vi "Change Current.vi"() -> ()   [LabVIEW 2011]
uses:
  <instrlib>/BK Precision 85XX Series/BK Precision 85XX Series.lvlib
panel:
  in  "CC Current (0)":dbl
  in  "VISA resource name":refnum<visa-resource-name>
  # "A"
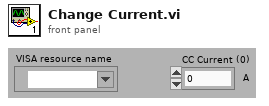
[diagram p1: front panel]
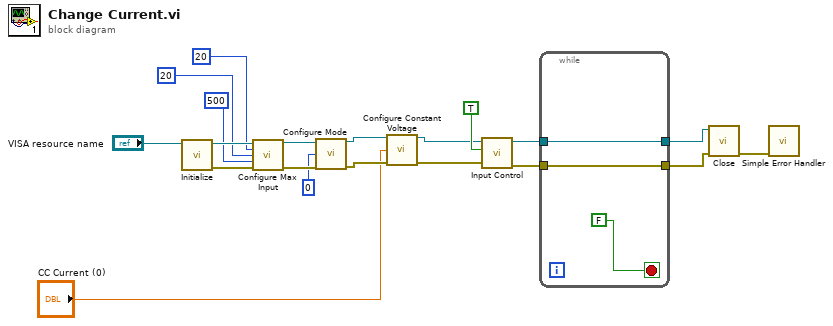
[diagram p0: block diagram]
diagram:
  n1 = call <instrlib>:"Initialize.vi"("VISA resource name"="VISA resource name") -> ("error out"=w20:errorcluster, "VISA resource name out"=w16:refnum<visa-resource-name>)  [unwired: 9 in]
  n2 = call <instrlib>:"Configure Max Input.vi"("VISA resource name"=w16, "Maximum Input Voltage (0)"=20, "Maximum Input Current (0)"=20, "Maximum Input Power (0)"=500, "error in (no error)"=w20) -> ("VISA resource name out"=w15:refnum<visa-resource-name>, "error out"=w19:errorcluster)  [unwired: 9 in]
  n3 = call <instrlib>:"Configure Mode.vi"("VISA resource name"=w15, "Mode of Operation (0:CC)"=0, "error in (no error)"=w19) -> ("VISA resource name out"=w12:refnum<visa-resource-name>, "error out"=w11:errorcluster)  [unwired: 11 in]
  n4 = call <instrlib>:"Configure Constant Voltage.vi"("VISA resource name"=w12, "CV Voltage (0)"="CC Current (0)", "error in (no error)"=w11) -> ("VISA resource name out"=w9:refnum<visa-resource-name>, "error out"=w10:errorcluster)  [unwired: 11 in]
  n5 = call <instrlib>:"Input Control.vi"("error in (no error)"=w10, "Enable Input Terminals (F: Off)"=TRUE, "VISA resource name"=w9) -> ("error out"=w1:errorcluster, "VISA resource name out"=w3:refnum<visa-resource-name>)  [unwired: 7 in]
  n6 = while {
    tunnel: [w23] -> w4
    tunnel: w3 -> [w23]
    tunnel: [w22] -> w2
    tunnel: w1 -> [w22]
    stop <- FALSE stop-if-true
  }
  n7 = call <instrlib>:"Close.vi"("error in (no error)"=w2, "VISA resource name"=w4) -> ("error out"=w14:errorcluster)  [unwired: 9 in]
  n8 = call <vilib>:"Simple Error Handler.vi"("error in (no error)"=w14) -> ()  [unwired: 4 in, 5 out]
